vi "rotate_calculate.vi"(10 "pieceOfWorld":T2[][](array[typedef]), 11 "input cluster":T1) -> (1 "angle":dbl, 2 "full round":bool, 3 "output cluster":T1)   [LabVIEW 2015, in "PolyVIEW.lvclass"]
uses:
  PolyVIEW.lvclass
  actors/world/typedefs/worldCell_cluster.ctl
  actors/world/typedefs/markValue_cluster.ctl
  actors/world/typedefs/markValue.ctl
  actors/world/typedefs/markVolume.ctl
  actors/world/typedefs/amountOfFood.ctl
  actors/world/typedefs/anthillType_enum.ctl
  Memory.ctl
  actors/world/world.lvlib
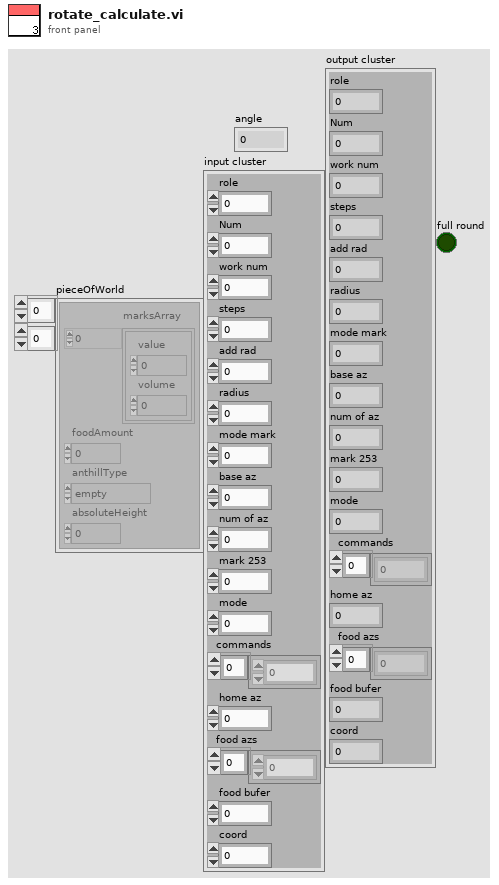
[diagram p1: front panel]
types:
  T1 = typedef "PolyVIEW.lvclass/Memory.ctl" = cluster{"role":i32, "Num":i32, "work num":i32, "steps":dbl, "add rad":i32, "radius":dbl, "mode mark":u32, "base az":dbl, "num of az":u32, "mark 253":u32, "mode":u32, "commands":i32[], "home az":dbl, "food azs":dbl[], "food bufer":dbl, "coord":cdb}
  T2 = typedef "world.lvlib/worldCell_cluster.ctl" = cluster{"marksArray":T3[], "foodAmount":T6, "anthillType":T7, "absoluteHeight":u8}
  T3 = typedef "world.lvlib/markValue_cluster.ctl" = cluster{"value":T4, "volume":T5}
  T4 = typedef "world.lvlib/markValue.ctl" = u8
  T5 = typedef "world.lvlib/markVolume.ctl" = u16
  T6 = typedef "world.lvlib/amountOfFood.ctl" = i32
  T7 = typedef "world.lvlib/anthillType_enum.ctl" = enum16{"empty", "own", "rival"}
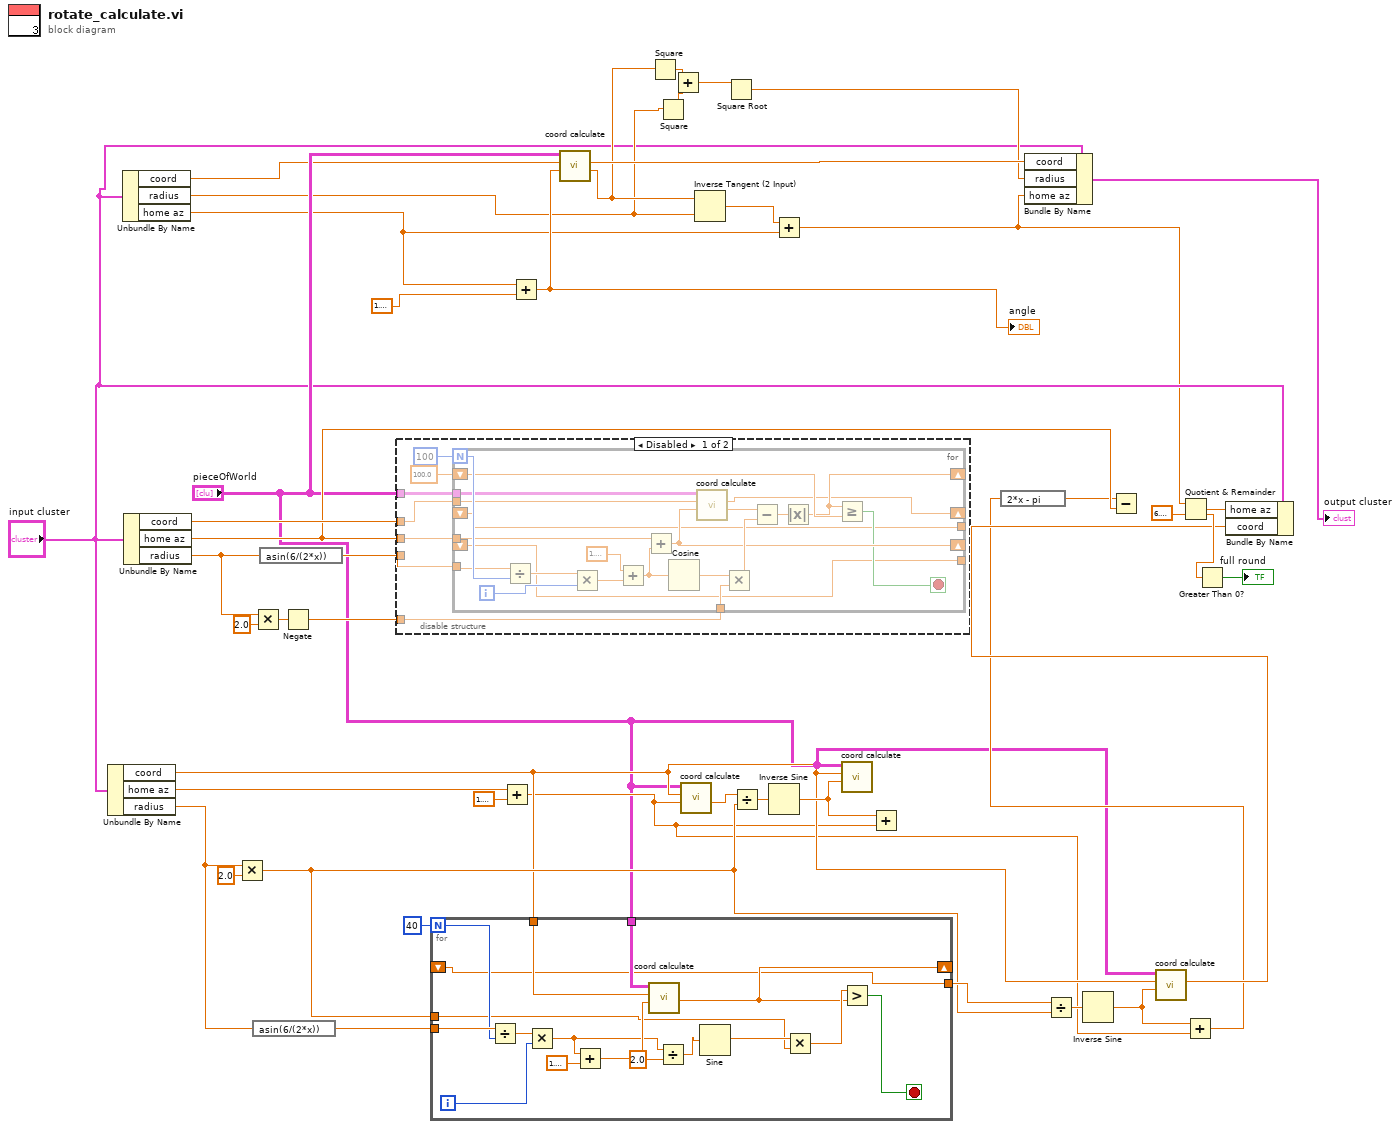
[diagram p0: block diagram]
diagram:
  n1 = Unbundle By Name("input cluster") -> ("coord"=w20:cdb, "home az"=w28:dbl, "radius"=w26:dbl)
  n2 = Unbundle By Name("input cluster") -> ("coord"=w14:cdb, "radius"=w7:dbl, "home az"=w10:dbl)
  n3 = Unbundle By Name("input cluster") -> ("coord"=w42:cdb, "home az"=w40:dbl, "radius"=w38:dbl)
  n4 = Multiply(x=w26, y=2.0) -> (x*y=w21:dbl)
  n5 = Multiply(x=w38, y=2.0) -> (x*y=w44:dbl)
  n6 = expression code="asin(6/(2*x))"(w26) -> (w25:dbl)
  n7 = expression code="asin(6/(2*x))"(w38) -> (w37:dbl)
  n8 = Negate(x=w44) -> (-x=w43:dbl)
  n9 = disable-structure shown="Disabled" {
    disable-tunnel: w43 -> [w50 _]
    disable-tunnel: w42 -> [w49 _]
    disable-tunnel: w40 -> [w48 _]
    disable-tunnel: w37 -> [w47 _]
    disable-tunnel: "pieceOfWorld" -> [w46 _]
    frame Disabled {
      n10 = for {
        N: 100 ("Numeric 5") -> [w72]
        tunnel: w50 -> [w73]
        tunnel: w46 -> [w69]
        shift-right: [w57] -> _
        shift-left: 100.0 ("Numeric 4") -> [w59]
        tunnel: w49 -> [w66]
        tunnel: w48 -> [w61]
        tunnel: w47 -> [w60]
        shift-right: [w65] -> _
        shift-left: _ -> [w56]
        tunnel: [w56] -> _
        shift-right: [w53] -> _
        shift-left: _ -> [w55]
        tunnel: [w55] -> _
        i -> [w71]
        stop <- w58 stop-if-true
        n11 = Divide(x=w60, y=w72) -> (x/y=w70:dbl)
        n12 = Multiply(x=w70, y=w71) -> (x*y=w63:dbl)
        n13 = Add(x=1.5707963267948966, y=w63) -> (x+y=w62:dbl)
        n14 = Add(x=w61, y=w62) -> (x+y=w65:dbl)
        n15 = Cosine(x=w62) -> (cos(x)=w74:dbl)
        n16 = call "coord calculate.vi"("theta"=w65, "coord in"=w66, "pieceOfWorld in"=w69) -> ("length"=w54:dbl, "coord out"=w53:cdb)  [unwired: 7 in]
        n17 = Multiply(x=w74, y=w73) -> (x*y=w68:dbl)
        n18 = Subtract(x=w54, y=w68) -> (x-y=w67:dbl)
        n19 = Absolute Value(x=w67) -> (abs(x)=w57:dbl)
        n20 = Greater Or Equal?(x=w57, y=w59) -> (x >= y?=w58:bool)
      }
    }
    frame Enabled {
    }
  }
  n21 = for {
    N: 40 -> [w90]
    tunnel: w25 -> [w91]
    tunnel: "pieceOfWorld" -> [w85]
    tunnel: w20 -> [w84]
    tunnel: w21 -> [w82]
    shift-right: [w76] -> _
    shift-left: _ -> [w75]
    tunnel: [w75] -> w22
    i -> [w88]
    stop <- w77 stop-if-true
    n22 = Divide(x=w91, y=w90) -> (x/y=w89:dbl)
    n23 = Multiply(x=w89, y=w88) -> (x*y=w81:dbl)
    n24 = Add(x=w81, y=1.5707963267948966) -> (x+y=w86:dbl)
    n25 = call "coord calculate.vi"("theta"=w86, "coord in"=w84, "pieceOfWorld in"=w85) -> ("length"=w76:dbl)  [unwired: 7 in, 1 out]
    n26 = Divide(x=w81, y=2.0) -> (x/y=w79:dbl)
    n27 = Sine(x=w79) -> (sin(x)=w83:dbl)
    n28 = Multiply(x=w83, y=w82) -> (x*y=w78:dbl)
    n29 = Greater?(x=w78, y=w76) -> (0:w77:bool)
  }
  n30 = Add(x=w28, y=1.5707963267948966) -> (x+y=w19:dbl)
  n31 = Add(x=w10, y=1.5707963267948966) -> (x+y=w13:dbl)
  "angle" <- w13
  n32 = call "coord calculate.vi"("theta"=w13, "coord in"=w14, "pieceOfWorld in"="pieceOfWorld") -> ("length"=w8:dbl, "coord out"=w12:cdb)  [unwired: 7 in]
  n33 = Square(x=w8) -> (x^2=w5:dbl)
  n34 = Square(x=w7) -> (x^2=w6:dbl)
  n35 = Add(x=w5, y=w6) -> (x+y=w9:dbl)
  n36 = call "coord calculate.vi"("theta"=w19, "coord in"=w20, "pieceOfWorld in"="pieceOfWorld") -> ("length"=w31:dbl)  [unwired: 7 in, 1 out]
  n37 = Inverse Tangent (2 Input)(1:w7, 2:w8) -> (0:w11:dbl)
  n38 = Square Root(x=w9) -> (sqrt(x)=w4:dbl)
  n39 = Divide(x=w31, y=w21) -> (x/y=w30:dbl)
  n40 = Inverse Sine(1:w30) -> (0:w29:dbl)
  n41 = Add(x=w11, y=w10) -> (x+y=w1:dbl)
  n42 = call "coord calculate.vi"("theta"=w29, "coord in"=w20, "pieceOfWorld in"="pieceOfWorld") -> ()  [unwired: 7 in, 2 out]
  n43 = Add(x=w29, y=w19) -> ()  [unwired: 1 out]
  n44 = Bundle By Name(cluster="input cluster", "coord"=w12, "radius"=w4, "home az"=w1) -> (→"output cluster":T1)
  n45 = Divide(x=w22, y=w21) -> (x/y=w24:dbl)
  n46 = Inverse Sine(1:w24) -> (0:w23:dbl)
  n47 = call "coord calculate.vi"("theta"=w23, "coord in"=w20, "pieceOfWorld in"="pieceOfWorld") -> ("coord out"=w18:cdb)  [unwired: 7 in, 1 out]
  n48 = Quotient & Remainder(x=w1, y=6.283185307179586) -> (x-y*floor(x/y)=w36:dbl, floor(x/y)=w35:dbl)
  n49 = Add(x=w23, y=w19) -> (x+y=w17:dbl)
  n50 = expression code="2*x - pi"(w17) -> (w39:dbl)
  n51 = Subtract(x=w39, y=w40) -> ()  [unwired: 1 out]
  n52 = Greater Than 0?(x=w35) -> (x > 0?=→"full round":bool)
  n53 = Bundle By Name(cluster="input cluster", "home az"=w36, "coord"=w18) -> ()  [unwired: 1 out]
